vi "SP Append Limit Waveform.vi"(4 "Limit Format":T2, 5 "Number of Points":i32, 6 "Measured Parameter":T3={"Stimulus Port"=1, "Response Port"=1} {"Stimulus Port" min=1 step=1; "Response Port" min=1 step=1}, 7 "Attribute Name (NI_ChannelName)":string="NI_ChannelName", 8 "error in (no error)":errorcluster, 9 "Limits Pass/Fail":cluster{"Upper Pass?":bool, "Lower Pass?":bool}, 10 "Upper and Lower Limits":T1={"Upper Limit"={"F0"=500.0, "dF"=1.0, "Formatted Values"=[-6.0, -6.0, -6.0, -6.0, -6.0, -6.0, -5.0, -4.0, -3.0, -2.0, -1.0017226002993769, -0.8636286738753696, -1.012432061728755, -0.8135188671805874, -1.084383696215112, -1.192695586219516, -0.8228939725524264, -1.1588169801015764, -1.0069715761898415, -0.8118111488159718, -0.9516999033989667, -1.0842662636672022, -1.0261931083967077, -0.816874162233468, -0.8335770068326294, -1.1794529347576463, -1.1032959879886735, -1.197742447623333, -0.9631229100196212, -0.9908453124177325, -0.9835470980893588, -1.10217991844936, -0.8956607286257672, -0.8794782872077156, -0.9013683651609963, -1.0772188731817596, -0.992723355191172, -0.9536275499498994, -0.9874327685983141, -0.921963653527827, -0.8848787728556787, -1.1874980208218, -0.996957511881206, -0.9972503730309241, -0.8866139538542095, -1.07344181331393, -0.881559772443858, -1.0112449407130875, -0.9865384477979471, -0.9901446738263366, -1.1718630063784758, -0.9951725256878827, -0.931778781153855, -0.9846289731021831, -0.851763264124267, -0.9086965469391421, -0.8349429101974368, -0.8383742350256687, -1.106571816484691, -0.9554005266395742, -0.9376822403043366, -1.131287512516927, -1.0382288806403288, -0.917054052988136, -0.9489467877812984, -0.9264227759143271, -1.0918690925892351, -1.1668737446636852, -1.0021735712381068, -1.1541225361979714, -1.1931131329605709, -0.8730502330378824, -0.850411285659811, -1.137775166801135, -1.1870586525662095, -1.0926571181161528, -1.118993526927924, -1.1211410787283602, -0.8920697041785735, -0.888430731015914, -1.0656600076605476, -1.1666787859795846, -1.0713340188424678, -0.8625910088884297, -1.1434360227216422, -0.9217710376784376, -1.1218396445954617, -0.9558195687190933, -1.1773692443654946, -1.0827782751424972, -1.1567791336122029, -0.8684407402614696, -0.8177845157195978, -0.9040657051180614, -0.9313557288389804, -1.0236831450620423, -1.050426714979035, -0.8344777069605718, -0.8274082929927138, -1.1990080831766776, -1.0947798998491134, -1.1963114865246718, -1.0016247375583676, -1.0877110100652403, -1.1556028882288836, -1.1918380581525247, -0.9751292214691399, -0.8884133044813358, -1.0347444321214612, -0.9445125246491541, -2.0, -3.0, -4.0, -5.0, -6.0, -6.0, -6.0, -6.0, -6.0, -6.0]}, "Lower Limit"={"F0"=500.0, "dF"=1.0, "Formatted Values"=[-6.0, -6.0, -6.0, -6.0, -6.0, -6.0, -5.0, -4.0, -3.0, -2.0, -1.0017226002993769, -0.8636286738753696, -1.012432061728755, -0.8135188671805874, -1.084383696215112, -1.192695586219516, -0.8228939725524264, -1.1588169801015764, -1.0069715761898415, -0.8118111488159718, -0.9516999033989667, -1.0842662636672022, -1.0261931083967077, -0.816874162233468, -0.8335770068326294, -1.1794529347576463, -1.1032959879886735, -1.197742447623333, -0.9631229100196212, -0.9908453124177325, -0.9835470980893588, -1.10217991844936, -0.8956607286257672, -0.8794782872077156, -0.9013683651609963, -1.0772188731817596, -0.992723355191172, -0.9536275499498994, -0.9874327685983141, -0.921963653527827, -0.8848787728556787, -1.1874980208218, -0.996957511881206, -0.9972503730309241, -0.8866139538542095, -1.07344181331393, -0.881559772443858, -1.0112449407130875, -0.9865384477979471, -0.9901446738263366, -1.1718630063784758, -0.9951725256878827, -0.931778781153855, -0.9846289731021831, -0.851763264124267, -0.9086965469391421, -0.8349429101974368, -0.8383742350256687, -1.106571816484691, -0.9554005266395742, -0.9376822403043366, -1.131287512516927, -1.0382288806403288, -0.917054052988136, -0.9489467877812984, -0.9264227759143271, -1.0918690925892351, -1.1668737446636852, -1.0021735712381068, -1.1541225361979714, -1.1931131329605709, -0.8730502330378824, -0.850411285659811, -1.137775166801135, -1.1870586525662095, -1.0926571181161528, -1.118993526927924, -1.1211410787283602, -0.8920697041785735, -0.888430731015914, -1.0656600076605476, -1.1666787859795846, -1.0713340188424678, -0.8625910088884297, -1.1434360227216422, -0.9217710376784376, -1.1218396445954617, -0.9558195687190933, -1.1773692443654946, -1.0827782751424972, -1.1567791336122029, -0.8684407402614696, -0.8177845157195978, -0.9040657051180614, -0.9313557288389804, -1.0236831450620423, -1.050426714979035, -0.8344777069605718, -0.8274082929927138, -1.1990080831766776, -1.0947798998491134, -1.1963114865246718, -1.0016247375583676, -1.0877110100652403, -1.1556028882288836, -1.1918380581525247, -0.9751292214691399, -0.8884133044813358, -1.0347444321214612, -0.9445125246491541, -2.0, -3.0, -4.0, -5.0, -6.0, -6.0, -6.0, -6.0, -6.0, -6.0]}}, 11 "Waveforms in":waveform(dbl)[](array[waveform])) -> (0 "error out":errorcluster, 3 "Waveforms out":waveform(dbl)[](array[waveform]))   [LabVIEW 2011]
uses:
  TypeDefs/SP Parameter.ctl
  TypeDefs/SP Format.ctl
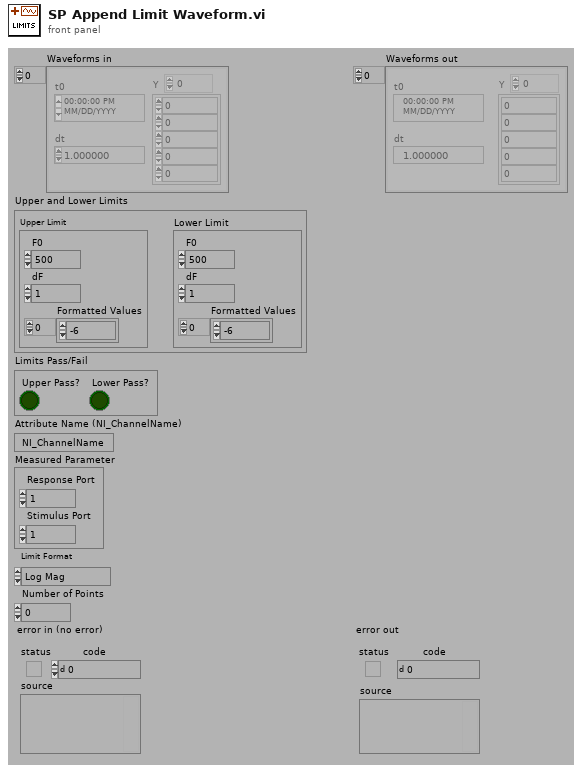
[diagram p1: front panel]
types:
  T1 = cluster{"Upper Limit":cluster{"F0":dbl, "dF":dbl, "Formatted Values":dbl[]}, "Lower Limit":cluster{"F0":dbl, "dF":dbl, "Formatted Values":dbl[]}}
  T2 = typedef "SP Format.ctl" = enum16{"Log Mag", "Lin Mag", "SWR", "Phase", "Expanded Phase", "Delay", "Insertion Loss", "Isolation", "Return Loss"}
  T3 = typedef "SP Parameter.ctl" = cluster{"Stimulus Port":i8, "Response Port":i8}
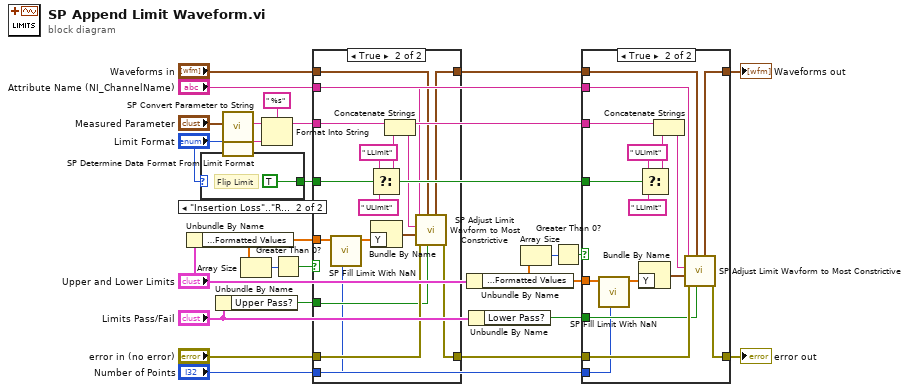
[diagram p0: block diagram]
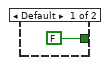
[diagram p2: hidden frame]
diagram:
  n1 = Unbundle By Name("Upper and Lower Limits") -> ("Upper Limit.Formatted Values"=w20:dbl[])
  n2 = case shown="\"Insertion Loss\"..\"Return Loss\"" "Limit Format" {
    tunnel: [FALSE TRUE] -> w5
    frame Default {
    }
    frame "Insertion Loss".."Return Loss" {
      # "Flip Limit"
    }
  }
  n3 = Unbundle By Name("Limits Pass/Fail") -> ("Upper Pass?"=w17:bool)
  n4 = call "SP Convert Parameter to String.vi"("Parameter"="Measured Parameter") -> ("Parameter String"=w2:string)  [unwired: 10 out]
  n5 = call "SP Determine Data Format From Limit Format.vi"("Limit Format"="Limit Format") -> ("Format String"=w3:string)
  n6 = Array Size(array=w20) -> (size(s)=w23:i32)
  n7 = Format Into String(format string=" %s", initial string=w2, w3) -> (resulting string=w13:string)  [unwired: 1 in, 1 out]
  n8 = Greater Than 0?(x=w23) -> (x > 0?=w21:bool)
  n9 = case shown="True" w21 {
    tunnel: "Waveforms in" -> [w28 w38]
    tunnel: "error in (no error)" -> [w29 w44]
    tunnel: [w29 w36] -> w10
    tunnel: "Attribute Name (NI_ChannelName)" -> [_ w34]
    tunnel: w20 -> [_ w32]
    tunnel: w13 -> [_ w43]
    tunnel: [w28 w37] -> w15
    tunnel: w17 -> [_ w35]
    tunnel: w5 -> [_ w39]
    tunnel: "Number of Points" -> [_ w30]
    frame False {
    }
    frame True {
      n10 = call "SP Fill Limit With NaN.vi"("Number of Points"=w30, "Limit"=w32) -> ("Filled Limit"=w31:dbl[])  [unwired: 9 out]
      n11 = Select(t=" LLimit", s=w39, f=" ULimit") -> (s? t:f=w40:string)
      n12 = Bundle By Name("Y"=w31) -> (w45:waveform(dbl))  [unwired: 1 out]
      n13 = Concatenate Strings(w43, w40) -> (w33:string)
      n14 = call "SP Adjust Limit Wavform to Most Constrictive.vi"("Pass?"=w35, "Waveforms In"=w38, "error in (no error)"=w44, "Waveform In"=w45, "Channel Name"=w33, "Attribute Name (NI_ChannelName)"=w34) -> ("error out"=w36:errorcluster, "Waveforms Out"=w37:waveform(dbl)[])  [unwired: 3 in, 1 out]
    }
  }
  n15 = Unbundle By Name("Upper and Lower Limits") -> ("Lower Limit.Formatted Values"=w8:dbl[])
  n16 = Unbundle By Name("Limits Pass/Fail") -> ("Lower Pass?"=w9:bool)
  n17 = Array Size(array=w8) -> (size(s)=w19:i32)
  n18 = Greater Than 0?(x=w19) -> (x > 0?=w7:bool)
  n19 = case shown="True" w7 {
    tunnel: w15 -> [w46 w55]
    tunnel: w10 -> [w47 w58]
    tunnel: [w47 w57] -> w11
    tunnel: "Attribute Name (NI_ChannelName)" -> [_ w54]
    tunnel: w8 -> [_ w50]
    tunnel: w13 -> [_ w63]
    tunnel: [w46 w56] -> w12
    tunnel: w9 -> [_ w51]
    tunnel: w5 -> [_ w59]
    tunnel: "Number of Points" -> [_ w48]
    frame False {
    }
    frame True {
      n20 = call "SP Fill Limit With NaN.vi"("Number of Points"=w48, "Limit"=w50) -> ("Filled Limit"=w49:dbl[])  [unwired: 9 out]
      n21 = Bundle By Name("Y"=w49) -> (w52:waveform(dbl))  [unwired: 1 out]
      n22 = Select(t=" ULimit", s=w59, f=" LLimit") -> (s? t:f=w60:string)
      n23 = Concatenate Strings(w63, w60) -> (w53:string)
      n24 = call "SP Adjust Limit Wavform to Most Constrictive.vi"("Pass?"=w51, "Waveforms In"=w55, "error in (no error)"=w58, "Waveform In"=w52, "Channel Name"=w53, "Attribute Name (NI_ChannelName)"=w54) -> ("error out"=w57:errorcluster, "Waveforms Out"=w56:waveform(dbl)[])  [unwired: 3 in, 1 out]
    }
  }
  "Waveforms out" <- w12
  "error out" <- w11
